vi "top_save_plots.vi"(8 "error in":errorcluster, 9 "Front_panel_refs":T1, 10 "Dynamic data":T2, 11 "Input parameters":T3={"Measurement type"=enum."Debug", "Sensor type"=enum."HPK_8in_256", "Identifier"="test.txt", "Open after execution?"=FALSE, "Plot after execution?"=FALSE, "Display channel"=0, "Voltage Delay (s)"=0.5, "Switch Delay (s)"=0.01, "VISA resource name source"="", "VISA resource name DMM"="", "VISA resource name LCR"="", "Compliance  Level (A)"=10.0, "Voltage Limit (V)"=1000.0, "Data storage location"="", "Scan voltages"="", "Use source as DMM?"=FALSE, "LCR signal frequenzy (Hz)"=10.0, "DMM device"=enum."Keithley2001", "Sampling number"=1, "Use env. sensors on"=enum."Sensirion sht1x/7x", "Switchboard Handle"=0, "Use Switchboard"=FALSE, "LCR signal voltage (V)"=10000.0, "Repeat"=1, "Scan voltages IV"="", "Scan voltages CV"="", "Hex pad numbers?"=FALSE, "Set measurement type"=enum."Debug", "Custom pad scan"="", "IV voltage Delay (s)"=0.5, "CV voltage Delay (s)"=0.5, "Needle measurement?"=FALSE, "Comments"="test.txt", "LCR signal frequenzy (kHz)"=10.0, "Compliance  Level (uA)"=10.0, "Open Correction Array"=array2304x3[6912 elements], "Current set voltage"=0.0, "Last set voltage"=0.0, "Current channel"=0, "Last OpenCorrection index"=-1, "Total curr/vltg every x steps"=10, "Current channel iteration"=0, "No CV corrections"=FALSE, "Mapfile"="", "Corrfile"="", "IV voltage file"=path "", "CV voltage file"=path "", "IV Switch Delay (s)"=0.01, "CV Switch Delay (s)"=0.01, "Invert polarity"=FALSE, "Set debug dirs"=FALSE, "Is n on p"=FALSE} {"CV Switch Delay (s)" format="%#_13g"; "IV Switch Delay (s)" format="%#_13g"; "Last set voltage" format="%#_13g"; "Current set voltage" format="%#_13g"; "CV voltage Delay (s)" format="%#_13g"; "IV voltage Delay (s)" format="%#_13g"; "Voltage Limit (V)" format="%#_13g"; "Voltage Delay (s)" format="%#_13g"; "Switch Delay (s)" format="%#_13g"}) -> (0 "error out":errorcluster, 1 "Front_panel_refs out":T1, 2 "Dynamic data out":T2, 3 "Input parameters out":T3={"Measurement type"=enum."Debug", "Sensor type"=enum."HPK_8in_256", "Identifier"="test.txt", "Open after execution?"=FALSE, "Plot after execution?"=FALSE, "Display channel"=0, "Voltage Delay (s)"=0.5, "Switch Delay (s)"=0.01, "VISA resource name source"="", "VISA resource name DMM"="", "VISA resource name LCR"="", "Compliance  Level (A)"=10.0, "Voltage Limit (V)"=1000.0, "Data storage location"="", "Scan voltages"="", "Use source as DMM?"=FALSE, "LCR signal frequenzy (Hz)"=10.0, "DMM device"=enum."Keithley2001", "Sampling number"=1, "Use env. sensors on"=enum."Sensirion sht1x/7x", "Switchboard Handle"=0, "Use Switchboard"=FALSE, "LCR signal voltage (V)"=10000.0, "Repeat"=1, "Scan voltages IV"="", "Scan voltages CV"="", "Hex pad numbers?"=FALSE, "Set measurement type"=enum."Debug", "Custom pad scan"="", "IV voltage Delay (s)"=0.5, "CV voltage Delay (s)"=0.5, "Needle measurement?"=FALSE, "Comments"="test.txt", "LCR signal frequenzy (kHz)"=10.0, "Compliance  Level (uA)"=10.0, "Open Correction Array"=array2304x3[6912 elements], "Current set voltage"=0.0, "Last set voltage"=0.0, "Current channel"=0, "Last OpenCorrection index"=-1, "Total curr/vltg every x steps"=10, "Current channel iteration"=0, "No CV corrections"=FALSE, "Mapfile"="", "Corrfile"="", "IV voltage file"=path "", "CV voltage file"=path "", "IV Switch Delay (s)"=0.01, "CV Switch Delay (s)"=0.01, "Invert polarity"=FALSE, "Set debug dirs"=FALSE, "Is n on p"=FALSE} {"CV Switch Delay (s)" format="%#_13g"; "IV Switch Delay (s)" format="%#_13g"; "Last set voltage" format="%#_13g"; "Current set voltage" format="%#_13g"; "CV voltage Delay (s)" format="%#_13g"; "IV voltage Delay (s)" format="%#_13g"; "Voltage Limit (V)" format="%#_13g"; "Voltage Delay (s)" format="%#_13g"; "Switch Delay (s)" format="%#_13g"})   [LabVIEW 2016]
doc: "Saves plots to disk."
uses:
  data_dynamic.ctl
  input_params.ctl
  refs_front_panel.ctl
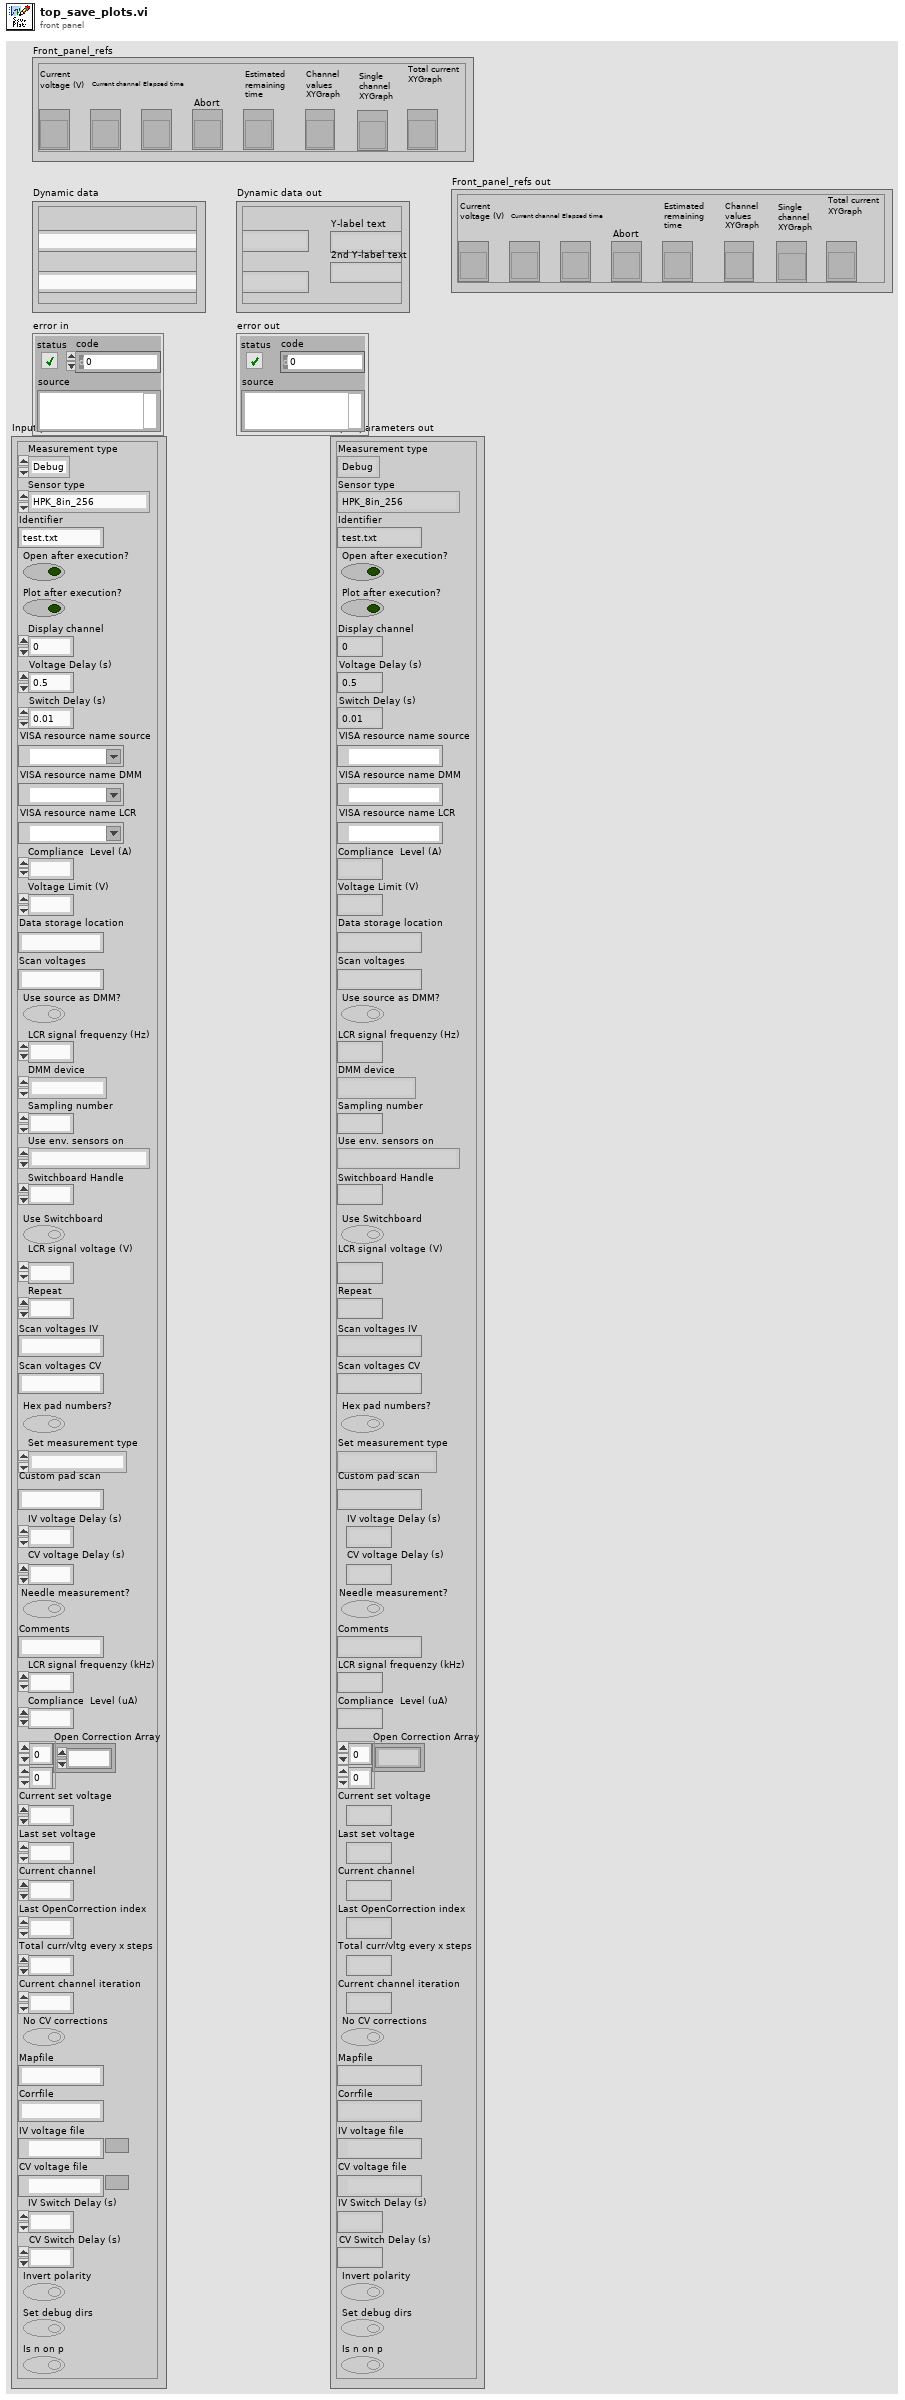
[diagram p1: front panel]
types:
  T1 = typedef "refs_front_panel.ctl" = cluster{"Current voltage (V)":refnum<vi>, "Elapsed time":refnum<vi>, "Current channel":refnum<vi>, "Abort":refnum<vi>, "Estimated remaining time":refnum<vi>, "Channel values XYGraph":refnum<vi>, "Single channel XYGraph":refnum<vi>, "Total current XYGraph":refnum<vi>}
  T2 = typedef "data_dynamic.ctl" = cluster{"Output file":path, "Y-label text":string, "Current set voltage":dbl, "Set voltage column":dbl[], "Pad number column":dbl[], "Data  column":dbl[], "Number of voltages":i32, "Compliance current (A)":dbl, "Geofile":string, "Peak voltage":dbl, "Hex PDF file":string, "Voltage array":dbl[], "Total current column":dbl[], "Timestamp column":dbl[], "Data name":string, "Data unit":string, "2nd data column":dbl[], "2nd data name":string, "2nd data unit":string, "3rd data column":dbl[], "4th data column":dbl[], "3rd data name":string, "3rd data unit":string, "4th data name":string, "4th data unit":string, "Actual voltage column":dbl[], "2nd Y-label text":string, "Single channel plot":path, "Temperature column":dbl[], "Humidity column":dbl[], "Channel switch array":i32[], "1st single plot name":string, "2nd single plot name":string, "All channels plot":path, "HexPlot command":string, "Custom channel array":i32[], "Data  error column":dbl[], "2nd data  error column":dbl[], "3rd data error column":dbl[], "4th data  error column":dbl[], "Total current plot":path, "5th data column":dbl[], "5th data  error column":dbl[], "6th data column":dbl[], "6th data  error column":dbl[], "5th data name":string, "5th data unit":string, "6th data name":string, "6th data unit":string, "HexPlot matrix command":string}
  T3 = typedef "input_params.ctl" = cluster{"Measurement type":enum16{"IV", "CV", "Debug", "Test_contact"}, "Sensor type":enum16{"HPK_6in_135", "HPK_8in_256", "IFX_8in_256", "Diode", "HPK_6in_256", "Full matrix"}, "Identifier":string, "Open after execution?":bool, "Plot after execution?":bool, "Display channel":i32, "Voltage Delay (s)":dbl, "Switch Delay (s)":dbl, "VISA resource name source":refnum<visa-resource-name>, "VISA resource name DMM":refnum<visa-resource-name>, "VISA resource name LCR":refnum<visa-resource-name>, "Compliance  Level (A)":dbl, "Voltage Limit (V)":dbl, "Data storage location":string, "Scan voltages":string, "Use source as DMM?":bool, "LCR signal frequenzy (Hz)":dbl, "DMM device":enum16{"Keithley2001", "Keithley2450", "Keithley2410", "Keithley6487"}, "Sampling number":i32, "Use env. sensors on":enum16{"Sensirion sht1x/7x", "Switch Matrix", "Probecard"}, "Switchboard Handle":u32, "Use Switchboard":bool, "LCR signal voltage (V)":dbl, "Repeat":i32, "Scan voltages IV":string, "Scan voltages CV":string, "Hex pad numbers?":bool, "Set measurement type":enum16{"IV", "CV", "Debug", "Test_contact", "IV+CV"}, "Custom pad scan":string, "IV voltage Delay (s)":dbl, "CV voltage Delay (s)":dbl, "Needle measurement?":bool, "Comments":string, "LCR signal frequenzy (kHz)":dbl, "Compliance  Level (uA)":dbl, "Open Correction Array":dbl[][], "Current set voltage":dbl, "Last set voltage":dbl, "Current channel":i32, "Last OpenCorrection index":i32, "Total curr/vltg every x steps":i32, "Current channel iteration":i32, "No CV corrections":bool, "Mapfile":string, "Corrfile":string, "IV voltage file":path, "CV voltage file":path, "IV Switch Delay (s)":dbl, "CV Switch Delay (s)":dbl, "Invert polarity":bool, "Set debug dirs":bool, "Is n on p":bool}
  T4 = typedef "imagedata.ctl" = cluster{"image type":i32, "image depth":i32, "image":u8[], "mask":u8[], "colors":u32[], "Rectangle":cluster{"left":i16, "top":i16, "right":i16, "bottom":i16}}
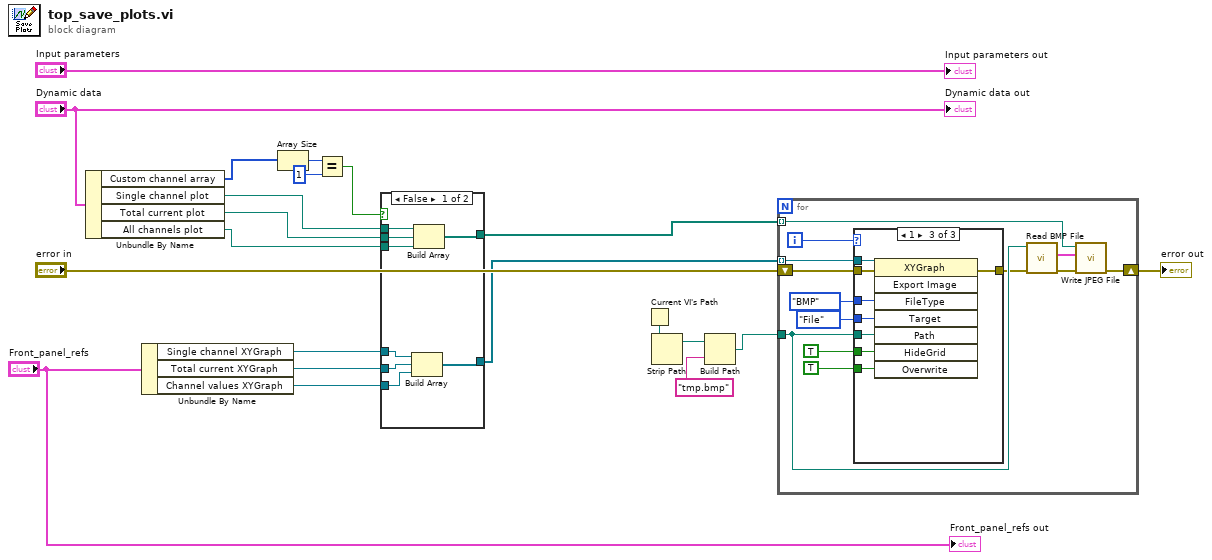
[diagram p0: block diagram]
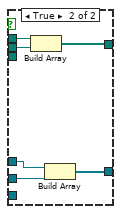
[diagram p2: hidden frame]
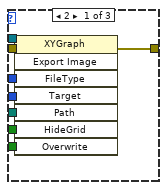
[diagram p3: hidden frame]
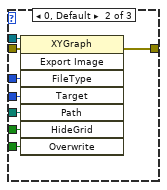
[diagram p4: hidden frame]
diagram:
  n1 = Unbundle By Name("Dynamic data") -> ("Custom channel array"=w13:i32[], "Single channel plot"=w17:path, "Total current plot"=w11:path, "All channels plot"=w10:path)
  n2 = Unbundle By Name("Front_panel_refs") -> ("Single channel XYGraph"=w4:refnum<vi>, "Total current XYGraph"=w3:refnum<vi>, "Channel values XYGraph"=w2:refnum<vi>)
  n3 = Array Size(array=w13) -> (size(s)=w15:i32)
  n4 = Equal?(x=w15, y=1) -> (x = y?=w12:bool)
  n5 = case shown="False" w12 {
    tunnel: w17 -> [w29 w35]
    tunnel: w10 -> [w28 _]
    tunnel: [w27 w34] -> w16
    tunnel: w11 -> [w26 w33]
    tunnel: w4 -> [w24 w32]
    tunnel: w3 -> [w25 w31]
    tunnel: w2 -> [w23 _]
    tunnel: [w22 w30] -> w1
    frame False {
      n6 = Build Array(w24, w25, w23) -> (w22:refnum<vi>[])
      n7 = Build Array(w29, w26, w28) -> (w27:path[])
    }
    frame True {
      n8 = Build Array(w35, w33) -> (w34:path[])
      n9 = Build Array(w32, w31) -> (w30:refnum<vi>[])
    }
  }
  n10 = Current VI's Path() -> (path=w21:path)
  n11 = Strip Path(path=w21) -> (stripped path=w18:path)  [unwired: 1 out]
  n12 = Build Path(base path=w18, name or relative path="tmp.bmp") -> (appended path=w19:path)
  n13 = for {
    tunnel: w19 -> [w48]
    shift-right: [w44] -> w7
    shift-left: "error in" -> [w43]
    tunnel: w16 -> [w42] mode=indexing
    tunnel: w1 -> [w40] mode=indexing
    i -> [w41]
    n14 = case shown="1" w41 {
      tunnel: enum32{"BMP", "EPS", "EMF", "PICT"}."BMP" ("File Type") -> [w52 w64 w70]
      tunnel: enum32{"File", "Clipboard"}."File" ("Target") -> [w53 w63 w69]
      tunnel: w48 -> [w54 w62 w68]
      tunnel: [w50 w61 w71] -> w47
      tunnel: TRUE ("Hide Grid") -> [w55 w60 w67]
      tunnel: TRUE ("Always Overwrite") -> [w56 w59 w66]
      tunnel: w43 -> [w51 w58 w72]
      tunnel: w40 -> [w49 w57 w65]
      frame 2 {
        n15 = invoke on="Invoke Node" class="XYGraph" method="Export Image"(reference=w49, error in=w51, "FileType"=w52, "Target"=w53, "Path"=w54, "HideGrid"=w55, "Overwrite"=w56) -> (error out=w50:errorcluster)  [unwired: 1 in, 7 out]
      }
      frame 0, Default {
        n16 = invoke on="Invoke Node" class="XYGraph" method="Export Image"(reference=w57, error in=w58, "FileType"=w64, "Target"=w63, "Path"=w62, "HideGrid"=w60, "Overwrite"=w59) -> (error out=w61:errorcluster)  [unwired: 1 in, 7 out]
      }
      frame 1 {
        n17 = invoke on="Invoke Node" class="XYGraph" method="Export Image"(reference=w65, error in=w72, "FileType"=w70, "Target"=w69, "Path"=w68, "HideGrid"=w67, "Overwrite"=w66) -> (error out=w71:errorcluster)  [unwired: 1 in, 7 out]
      }
    }
    n18 = call <vilib>:"Read BMP File.vi"("error in (no error)"=w47, "path to BMP file"=w48) -> ("error out"=w45:errorcluster, "image data"=w46:T4)  [unwired: 7 in, 1 out]
    n19 = call <vilib>:"Write JPEG File.vi"("error in (no error)"=w45, "image data"=w46, "path to JPEG file"=w42) -> ("error out"=w44:errorcluster)  [unwired: 7 in, 1 out]
  }
  "error out" <- w7
  "Input parameters out" <- "Input parameters"
  "Dynamic data out" <- "Dynamic data"
  "Front_panel_refs out" <- "Front_panel_refs"
